vi "Flatten.vi"(8 "error in":errorcluster, 9 "Data":T1) -> (0 "error out":errorcluster, 2 "Buffer":u8[](array[numeric]) format="%.0x")   [LabVIEW 2020, in "TcpReply.lvlib"]
uses:
  TcpReply.lvlib
  Data.ctl
  <vilib>/IlluminatedG/IG Protoc/LV-Proto/Wire Encode Tag.vi
  <vilib>/IlluminatedG/IG Protoc/LV-Proto/Encode LEN.vi
  <vilib>/IlluminatedG/IG Protoc/LV-Proto/Wire Encode Varint I32.vi
  <vilib>/IlluminatedG/IG Protoc/LV-Proto/LV-Proto.lvlib
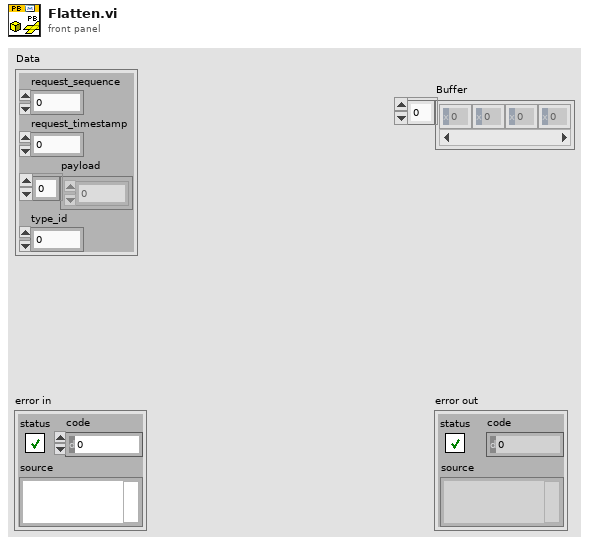
[diagram p1: front panel]
types:
  T1 = typedef "TcpReply.lvlib/Data.ctl" = cluster{"request_sequence":u32, "request_timestamp":u64, "payload":u8[], "type_id":u32}
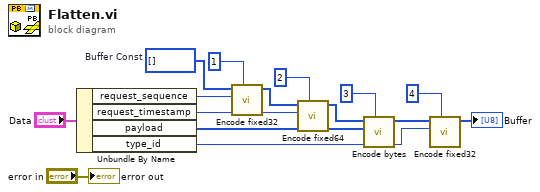
[diagram p0: block diagram]
diagram:
  w13 = u8[] []  # Buffer Const
  n1 = Unbundle By Name("Data") -> ("request_sequence"=w11:u32, "request_timestamp"=w8:u64, "payload"=w5:u8[], "type_id"=w2:u32)
  n2 = call <vilib>:"Encode fixed32.vi"("Field Number"=1, "fixed32"=w11, "Buffer in"=w13) -> ("Buffer"=w10:u8[])  [unwired: 8 in]
  n3 = call <vilib>:"Encode fixed64.vi"("Field Number"=2, "fixed64"=w8, "Buffer in"=w10) -> ("Buffer"=w7:u8[])  [unwired: 8 in]
  n4 = call <vilib>:"Encode bytes.vi"("Field Number"=3, "bytes"=w5, "Buffer in"=w7) -> ("Buffer"=w4:u8[])  [unwired: 8 in]
  n5 = call <vilib>:"Encode fixed32.vi"("Field Number"=4, "fixed32"=w2, "Buffer in"=w4) -> ("Buffer"=→"Buffer":u8[])  [unwired: 8 in]
  "error out" <- "error in"
